vi "Ideal_pulse.vi"(9 "Sensitivity":dbl, 10 "Amplitude":dbl, 11 "Length":dbl) -> (3 "Cluster":cluster{dbl, dbl, "Sinusoidal Pattern":dbl[]})   [LabVIEW 2020]
uses:
  <vilib>/Analysis/NI_AALBase.lvlib
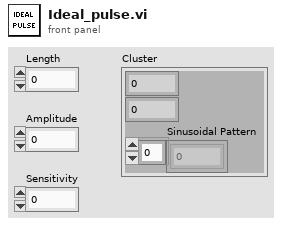
[diagram p1: front panel]
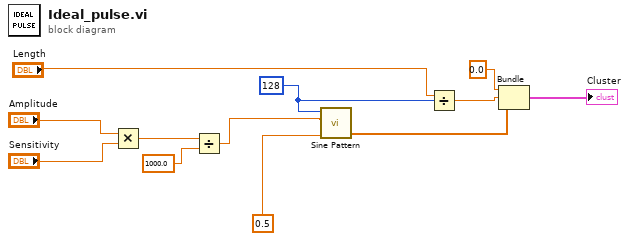
[diagram p0: block diagram]
diagram:
  w10 = 128 ("samples")
  n1 = Multiply(x="Amplitude", y="Sensitivity") -> (x*y=w3:dbl)
  n2 = Divide(x=w3, y=1000.0) -> (x/y=w1:dbl)
  n3 = call <vilib>:"Sine Pattern.vi"("cycles"=0.5, "amplitude"=w1, "samples"=w10) -> ("Sinusoidal Pattern"=w7:dbl[])  [unwired: 1 in, 1 out]
  n4 = Divide(x="Length", y=w10) -> (x/y=w11:dbl)
  n5 = Bundle(0.0, w11, "Sinusoidal Pattern"=w7) -> (→"Cluster":cluster{dbl, dbl, "Sinusoidal Pattern":dbl[]})  [unwired: 1 in]
